vi "DraggingDresser.vi"() -> ()   [LabVIEW 2014]
panel:
  out "Force":dbl[](array[numeric])
  out "Angle for Minimum Force":i32 format="%.1f"
  in  "Coefficient of Kinetic Friction":dbl format="%.1f"
  out "Waveform Graph":dbl[](graph)
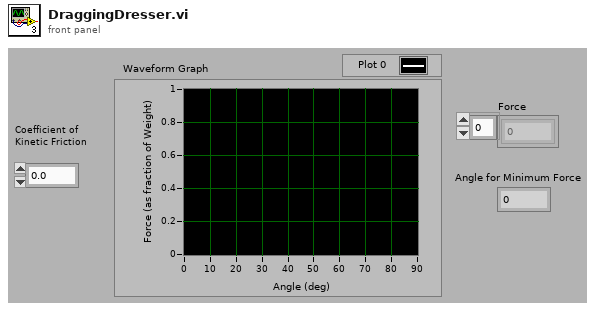
[diagram p1: front panel]
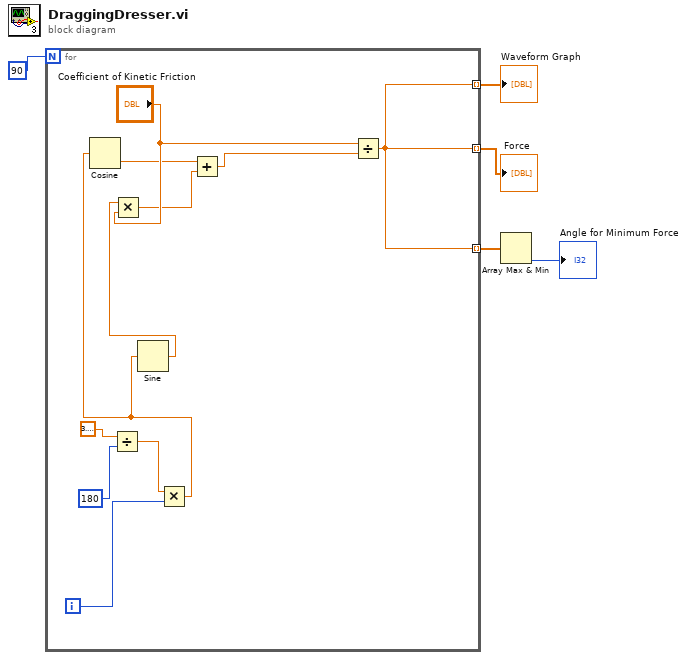
[diagram p0: block diagram]
diagram:
  n1 = for {
    N: 90 -> [_]
    tunnel: [w12] -> w5 mode=indexing
    tunnel: [w12] -> w4 mode=indexing
    tunnel: [w12] -> w2 mode=indexing
    i -> [w9]
    n2 = Divide(x=3.141592653589793, y=180) -> (x/y=w8:dbl)
    n3 = Multiply(x=w8, y=w9) -> (x*y=w6:dbl)
    n4 = Cosine(x=w6) -> (cos(x)=w14:dbl)
    n5 = Sine(x=w6) -> (sin(x)=w7:dbl)
    n6 = Multiply(x=w7, y="Coefficient of Kinetic Friction") -> (x*y=w15:dbl)
    n7 = Add(x=w14, y=w15) -> (x+y=w13:dbl)
    n8 = Divide(x="Coefficient of Kinetic Friction", y=w13) -> (x/y=w12:dbl)
  }
  "Waveform Graph" <- w4
  "Force" <- w5
  n9 = Array Max & Min(array=w2) -> (min index (indices)=→"Angle for Minimum Force":i32)  [unwired: 3 out]
